vi "fuzzy1.vi"() -> ()   [LabVIEW 2019]
uses:
  <vilib>/addons/Fuzzy Logic/FL Fuzzy Controller (MISO).vi
  <vilib>/addons/Fuzzy Logic/NI_Fuzzy_Logic_API.lvlib
panel:
  in  "file path":path
  out "Waveform Chart":T1(graph)
  in  "Set point":dbl
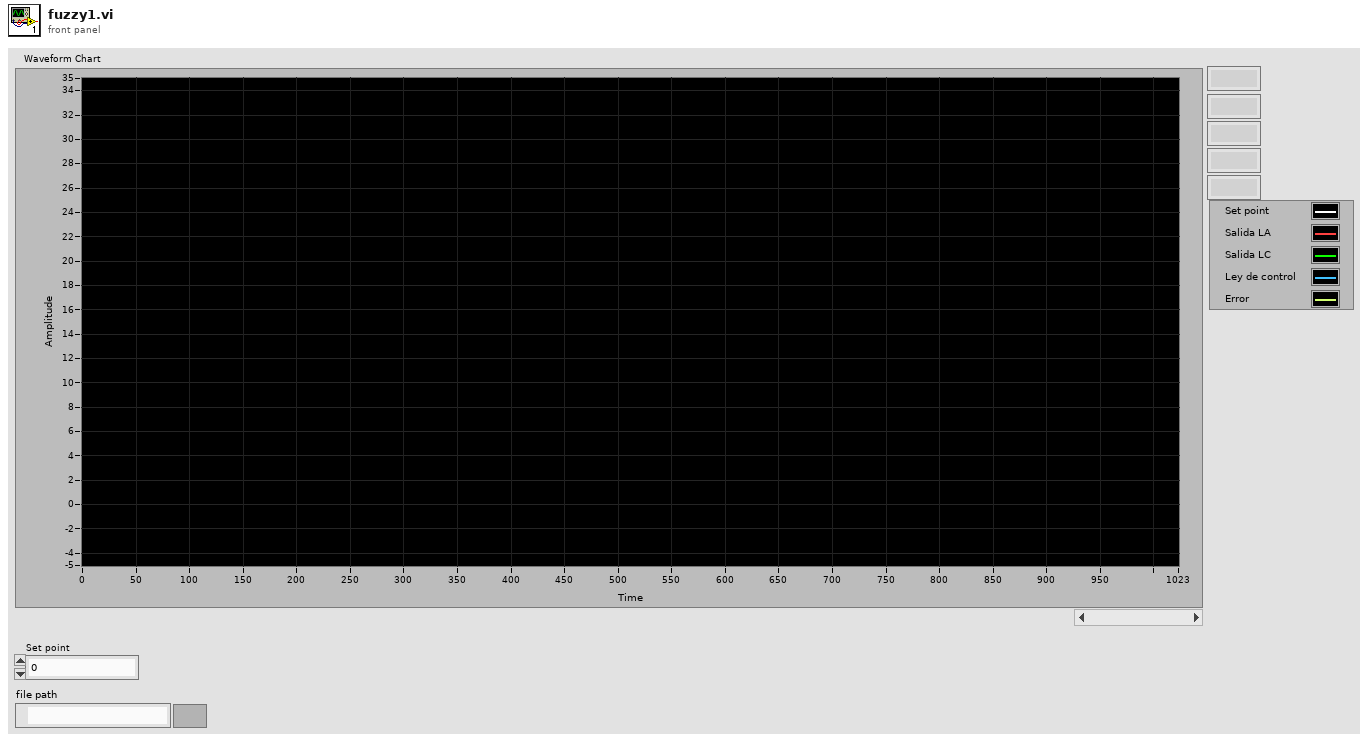
[diagram p1: front panel]
types:
  T1 = cluster{"Valvula (u_k)":dbl, "y_k":dbl, "y_k":dbl, "output value":dbl, dbl}
  T2 = typedef "NI_Fuzzy_Logic_API.lvlib/FL System.ctl" = cluster{"input variables":T3[], "output variables":T3[], "rules":T6[], "defuzzification method":T12, "description":string, "user MF interpolating polynomials":T13[]}
  T3 = typedef "NI_Fuzzy_Logic_API.lvlib/FL Variable.ctl" = cluster{"name":string, "range":dbl[], "MFs":T4[]}
  T4 = typedef "NI_Fuzzy_Logic_API.lvlib/FL Membership Function.ctl" = cluster{"name":string, "shape":T5, "points":dbl[], "color":u32, "user-defined shape index":i32}
  T5 = typedef "NI_Fuzzy_Logic_API.lvlib/FL Membership Function Shape.ctl" = u16
  T6 = typedef "NI_Fuzzy_Logic_API.lvlib/FL Rule.ctl" = cluster{"antecedents":T7[], "antecedent connective":T9, "consequents":T10[], "consequent implication":T11, "degree of support":dbl}
  T7 = typedef "NI_Fuzzy_Logic_API.lvlib/FL Antecedent.ctl" = cluster{"Var Index":i32, "MF Index":i32, "Cond":T8}
  T8 = typedef "NI_Fuzzy_Logic_API.lvlib/FL Modifier.ctl" = u16
  T9 = typedef "NI_Fuzzy_Logic_API.lvlib/FL Antecedent Connective.ctl" = u16
  T10 = typedef "NI_Fuzzy_Logic_API.lvlib/FL Consequent.ctl" = cluster{"Var Index":i32, "MF Index":i32, "Cond":T8}
  T11 = typedef "NI_Fuzzy_Logic_API.lvlib/FL Consequent Implication.ctl" = u16
  T12 = typedef "NI_Fuzzy_Logic_API.lvlib/FL Defuzzification.ctl" = u16
  T13 = typedef "NI_Fuzzy_Logic_API.lvlib/FL Interpolating polynomials.ctl" = cluster{"X":dbl[], "Y":dbl[], "Y(x) coeff":dbl[][], "X(y) coeff":dbl[][], "Area(y) coeff":dbl[][], "coa_x(y) coeff":dbl[][]}
  T14 = cluster{"Set point":dbl, "y_k":dbl, "y_k":dbl, "output value":dbl, dbl}
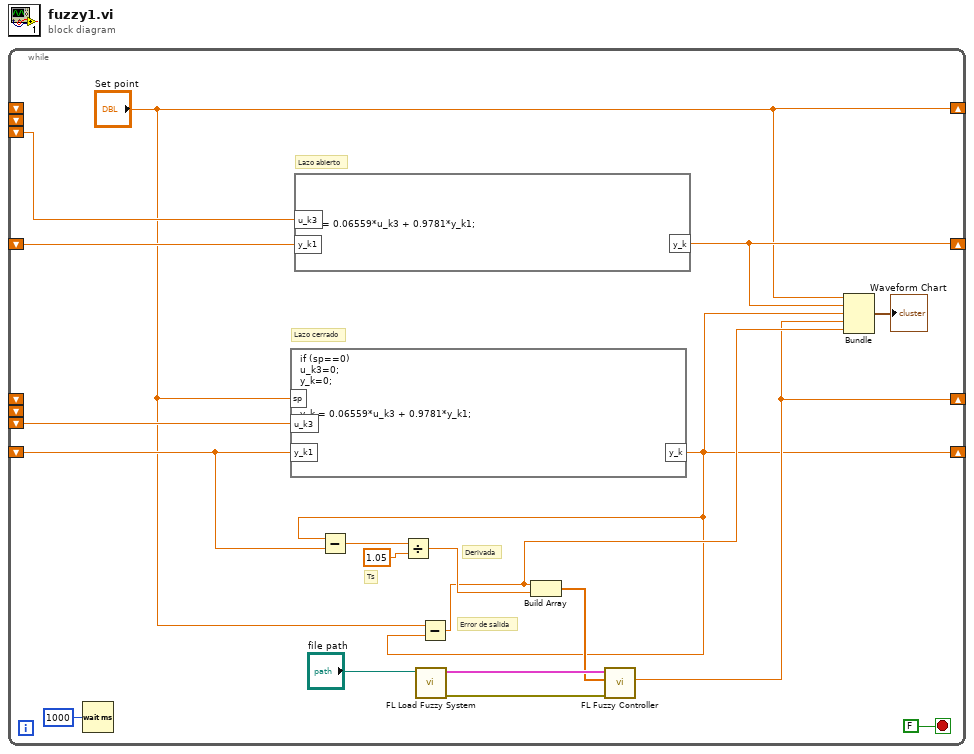
[diagram p0: block diagram]
diagram:
  n1 = while {
    shift-right: ["Set point"] -> _
    shift-left: _ -> [_]
    shift-left: _ -> [_]
    shift-left: _ -> [w19]
    shift-right: [w16] -> _
    shift-left: _ -> [w18]
    shift-right: [w1] -> _
    shift-left: _ -> [w9]
    shift-right: [w2] -> _
    shift-left: _ -> [_]
    shift-left: _ -> [_]
    shift-left: _ -> [w7]
    stop <- FALSE stop-if-true
    # "Lazo cerrado"
    # "Lazo abierto"
    # "Ts"
    # "Error de salida"
    # "Derivada"
    n2 = Wait (ms)(milliseconds to wait=u32 1000) -> ()  [unwired: 1 out]
    n3 = formula code="if (sp==0)\nu_k3=0;\ny_k=0;\n\n\ny_k = 0.06559*u_k3 + 0.9781*y_k1;\n\n\n\n\n\n\n\n\n\n\n\n\n\n\n\n\n\n\n\n\n\nif (sp==10)\ny_k = (0.06559*u_k3 + 0.9781*y_k1)*0.9951;"("u_k3"=w7, "y_k1"=w9, "sp"="Set point") -> ("y_k"=w1:dbl)
    n4 = formula code="y_k = 0.06559*u_k3 + 0.9781*y_k1;"("u_k3"=w19, "y_k1"=w18) -> ("y_k"=w16:dbl)
    n5 = Subtract(x=w1, y=w9) -> (x-y=w11:dbl)
    n6 = Divide(x=w11, y=1.05) -> (x/y=w5:dbl)
    n7 = call <vilib>:"FL Load Fuzzy System.vi"("file path"="file path") -> ("error out"=w12:errorcluster, "fuzzy system out"=w13:T2)  [unwired: 9 in]
    n8 = Subtract(x="Set point", y=w1) -> (x-y=w3:dbl)
    n9 = Build Array(w3, w5) -> (w8:dbl[])
    n10 = call-poly <vilib>:"FL Fuzzy Controller.vi"("error in (no error)"=w12, "input values"=w8, "fuzzy system in"=w13) -> ("output value"=w2:dbl)  [unwired: 4 in, 4 out]
    n11 = Bundle("Set point"="Set point", "y_k"=w16, "y_k"=w1, "output value"=w2, w3) -> (→"Waveform Chart":T14)  [unwired: 1 in]
  }
